vi "Create EventsLog Q.vi"(8 "error in (no error)":errorcluster, 10 "EventLog":T1, 11 "QName":string) -> (0 "error out":errorcluster, 3 "EventLogDataQRef":refnum<queue>)   [LabVIEW 2020]
doc: "Developed by Kevin Thompson\nThompson Engineering, LLC\nkevin@thompsonengineering.net"
uses:
  GBL DataQ Ref.vi
  TD EventLogData--cluster.ctl
panel:
  out "data reference":u32
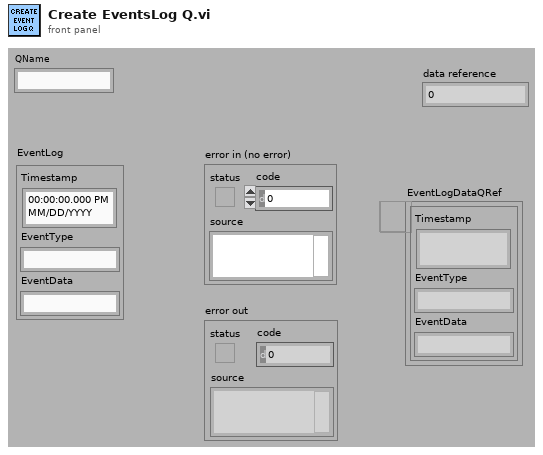
[diagram p1: front panel]
types:
  T1 = typedef "TD EventLogData--cluster.ctl" = cluster{"Timestamp":timestamp, "EventType":string, "EventData":string}
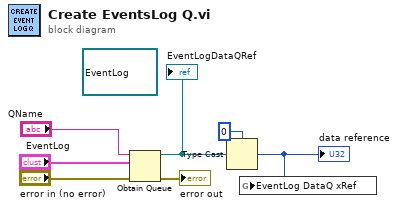
[diagram p0: block diagram]
diagram:
  (unwired) refnum<queue> refnum ("EventLogDataQRef")
  n1 = Obtain Queue(name (unnamed)="QName", element data type="EventLog", error in (no error)="error in (no error)") -> (queue out=w1:refnum<queue>, error out=→"error out":errorcluster)  [unwired: 2 in, 1 out]
  "EventLogDataQRef" <- w1
  n2 = Type Cast(type=u32 0, x=w1) -> (*(type *) &x=w3:u32)
  "data reference" <- w3
  n3 = global write "GBL DataQ Ref.vi" "EventLog DataQ xRef"(w3) -> ()
